vi "Decompose Command String.vi"(8 "Error In":errorcluster, 11 "Command IN":string) -> (0 "Error Out":errorcluster, 2 "ArgumentTable":string[][](array[string]), 3 "Action":string)   [LabVIEW 2012]
uses:
  <vilib>/regexp/Match Regular Expression.xnode
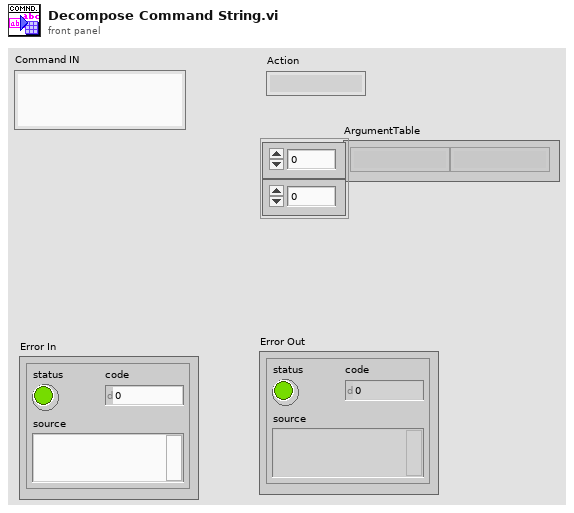
[diagram p1: front panel]
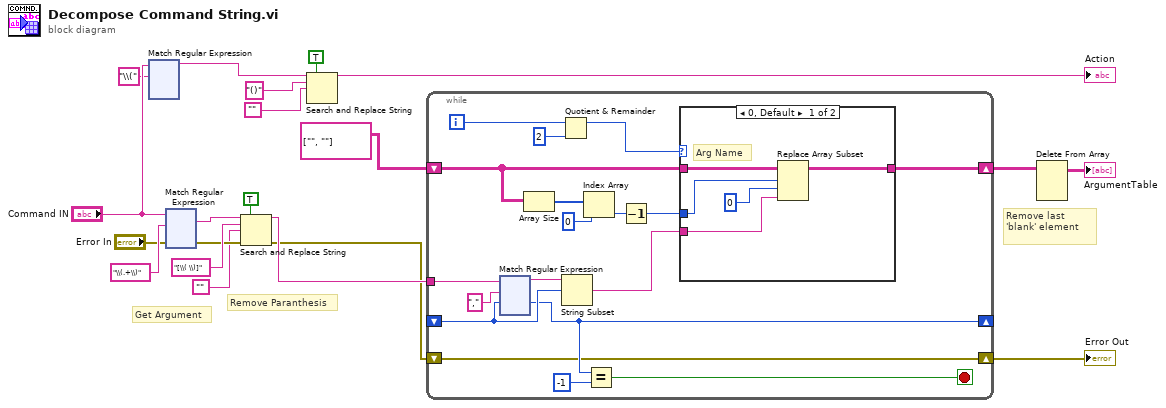
[diagram p0: block diagram]
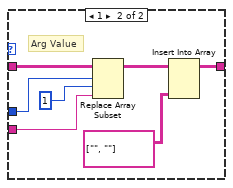
[diagram p2: hidden frame]
diagram:
  # "Remove last 'blank' element"
  # "Get Argument"
  # "Remove Paranthesis"
  n1 = xnode "Match Regular Expression"("input string"="Command IN", "regular expression"="\\(") -> ("before match"=w1:string)  [unwired: 4 in, 4 out]
  n2 = xnode "Match Regular Expression"("input string"="Command IN", "regular expression"="\\(.+\\)" ("search string/char (-)"), "error in"="Error In") -> ("whole match"=w5:string, "error out"=w18:errorcluster)  [unwired: 3 in, 3 out]
  n3 = Search and Replace String(replace all?=TRUE ("replace all? (F)"), input string=w5, search string="[\\( \\)]", replace string="", error in=w18) -> (result string=w8:string, error out=w6:errorcluster)  [unwired: 3 in, 2 out]
  n4 = Search and Replace String(replace all?=TRUE ("replace all? (F)"), input string=w1, search string="()", replace string="") -> (result string=→"Action":string)  [unwired: 4 in, 3 out]
  n5 = while {
    tunnel: w8 -> [w37]
    shift-right: [w30] -> _
    shift-left: _ -> [w35]
    shift-right: [w25] -> w14
    shift-left: string[][] [["", ""]] -> [w22]
    shift-right: [w21] -> w12
    shift-left: w6 -> [w21]
    i -> [w34]
    stop <- w28 stop-if-true
    n6 = xnode "Match Regular Expression"("input string"=w37, "regular expression"="," ("search string/char (-)"), "offset (0)"=w35) -> ("before match"=w36:string, "offset past match"=w30:i32)  [unwired: 3 in, 3 out]
    n7 = Array Size(array=w22) -> (size(s)=w27:i32[])
    n8 = Quotient & Remainder(x=w34, y=2) -> (x-y*floor(x/y)=w32:i32)  [unwired: 1 out]
    n9 = String Subset(string=w36, offset (0)=w35) -> (substring=w31:string)  [unwired: 1 in]
    n10 = Index Array(array=w27, index=0) -> (element=w24:i32)
    n11 = Equal?(x=w30, y=-1) -> (x = y?=w28:bool)
    n12 = Decrement(x=w24) -> (x-1=w23:i32)
    n13 = case shown="0, Default" w32 {
      tunnel: w31 -> [w40 w47]
      tunnel: [w39 w44] -> w25
      tunnel: w22 -> [w42 w50]
      tunnel: w23 -> [w41 w49]
      frame 0, Default {
        # "Arg Name"
        n14 = Replace Array Subset(array=w42, new element=w40, index (row)=w41, index (col)=0 ("disabled index (col)")) -> (w39:string[][])
      }
      frame 1 {
        # "Arg Value"
        n15 = Replace Array Subset(array=w50, new element=w47, index (row)=w49, index (col)=1 ("disabled index (col)")) -> (w45:string[][])
        n16 = Insert Into Array(array=w45, new element=string[][] [["", ""]]) -> (w44:string[][])  [unwired: 2 in]
      }
    }
  }
  "Error Out" <- w12
  n17 = Delete From Array "Delete From Array"(array=w14) -> (array with subset deleted=→"ArgumentTable":string[][])  [unwired: 3 in, 1 out]
